vi "Dispose Notification Icon.vi"(0 "NotifyIcon in":refnum<class "NotifyIcon.lvclass">, 11 "error in (no error)":errorcluster) -> (15 "error out":errorcluster)   [LabVIEW 2016, in "NotifyIcon.lvclass"]
doc: "This VI deletes the NotifyIcon Class instance and disposes all contained references and events.\n\nDynamically registered user events should be unregistered prior to calling this VI.\n\n\nStinus Olsen\nCIM Industrial Systems A/S\n22. Feb. 2011 15:04\nmailto: seo@cim.as"
uses:
  NotifyIcon.lvclass
  NotifyIcon.lvclass/NotifyIcon.ctl
  System.Windows.Forms
panel:
  # "This VI belongs to the NotifyIcon Toolset. \nA toolset that makes it easy to create, control and manipulate a notification icon in the notification area of the Windows taskbar.\nThe toolset requires Microsoft .NET framework 2.0\n\n\nNOTICE -- YOU MUST LEAVE THIS NOTICE IN PLACE.  PER THE TERMS OF THE LICENSE BELOW, YOU MAY SUBLICENSE THIS SOFTWARE \nIN ANY WAY THAT DOES NOT CONFLICT WITH THIS LICENSE.\n\n### BSD License (http://www.opensource.org/licenses/bsd-license.php) Begin ###\n \nCopyright (c) 2011, Stinus Olsen <seo@cim.as>\n\nAll rights reserved.\n\nRedistribution and use in source and binary forms, with or without modification, are permitted provided that the following conditions are met:\n\n    * Redistributions of source code must retain the above copyright notice, this list of conditions and the following disclaimer.\n    * Redistributions in binary form must reproduce the above copyright notice, this list of conditions and the following disclaimer in the \n       documentation and/or other materials provided with the distribution.\n    * Neither the name of CIM Industrial Systems nor the names of its contributors may be used to endorse or promote products derived \n       from this software without specific prior written permission.\n\nTHIS SOFTWARE IS PROVIDED BY THE COPYRIGHT HOLDERS AND CONTRIBUTORS \"AS IS\" AND ANY EXPRESS OR IMPLIED WARRANTIES, \nINCLUDING, BUT NOT LIMITED TO, THE IMPLIED WARRANTIES OF MERCHANTABILITY AND FITNESS FOR A PARTICULAR PURPOSE ARE \nDISCLAIMED. IN NO EVENT SHALL THE COPYRIGHT OWNER OR CONTRIBUTORS BE LIABLE FOR ANY DIRECT, INDIRECT, INCIDENTAL,\n SPECIAL, EXEMPLARY, OR CONSEQUENTIAL DAMAGES (INCLUDING, BUT NOT LIMITED TO, PROCUREMENT OF SUBSTITUTE GOODS OR \nSERVICES; LOSS OF USE, DATA, OR PROFITS; OR BUSINESS INTERRUPTION) HOWEVER CAUSED AND ON ANY THEORY OF LIABILITY, \nWHETHER IN CONTRACT, STRICT LIABILITY, OR TORT (INCLUDING NEGLIGENCE OR OTHERWISE) ARISING IN ANY WAY OUT OF THE USE \nOF THIS SOFTWARE, EVEN IF ADVISED OF THE POSSIBILITY OF SUCH DAMAGE.\n\n### BSD License End ###"
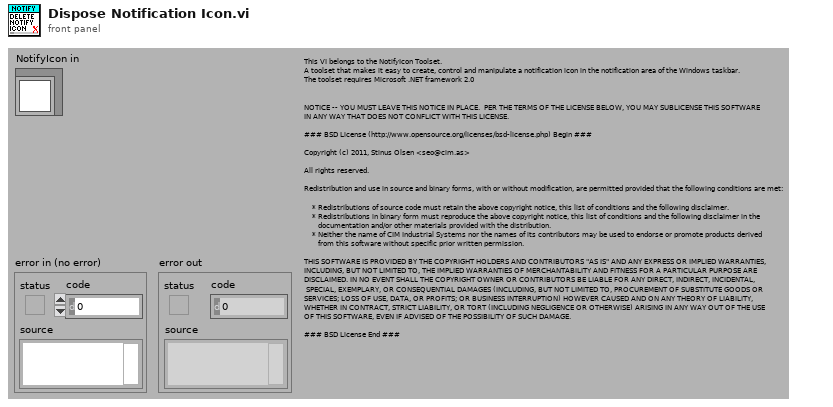
[diagram p1: front panel]
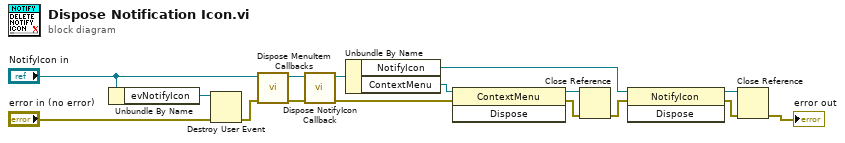
[diagram p0: block diagram]
diagram:
  n1 = Unbundle By Name("NotifyIcon in") -> ("evNotifyIcon"=w11:refnum<user-event>)
  n2 = Destroy User Event(user event=w11, error in="error in (no error)") -> (error out=w10:errorcluster)
  n3 = call "Dispose MenuItem Callbacks.vi"("error in (no error)"=w10, "NotifyIcon in"="NotifyIcon in") -> ("error out"=w8:errorcluster, "NotifyIcon out"=w9:refnum<class "NotifyIcon.lvclass">)  [unwired: 8 out]
  n4 = call "Dispose NotifyIcon Callback.vi"("error in (no error)"=w8, "NotifyIcon in"=w9) -> ("error out"=w1:errorcluster, "NotifyIcon out"=w7:refnum<class "NotifyIcon.lvclass">)  [unwired: 8 out]
  n5 = Unbundle By Name(w7) -> ("NotifyIcon"=w2:refnum<k24>, "ContextMenu"=w4:refnum<k24>)
  n6 = invoke class="ContextMenu" method="Dispose"(reference=w4, error in=w1) -> (reference out=w6:refnum<k24>, error out=w5:errorcluster)  [unwired: 1 in, 1 out]
  n7 = Close Reference(reference=w6, error in (no error)=w5) -> (error out=w3:errorcluster)
  n8 = invoke class="NotifyIcon" method="Dispose"(reference=w2, error in=w3) -> (reference out=w12:refnum<k24>, error out=w13:errorcluster)  [unwired: 1 in, 1 out]
  n9 = Close Reference(reference=w12, error in (no error)=w13) -> (error out=→"error out":errorcluster)
